vi "Panel.vi"(11 "StringPanel in":refnum<class "StringPanel.lvclass">) -> ()   [LabVIEW 2020, in "Conditum-Tools.lvlib" / "StringPanel.lvclass"]
uses:
  StringPanel.lvclass
  C:/dev/lv20CE/lv-conditum-tools/Conditum-Tools/ColumnPanel/ColumnPanel.lvclass
  C:/Program Files (x86)/National Instruments/LabVIEW 2020/vi.lib/IlluminatedG/IG OOPanel/OOPanel/Panel/Panel.lvclass
  ColumnPanel/Common Items.ctl
  <vilib>/IlluminatedG/IG OOPanel/OOPanel/Panel/Basic UI State.ctl
  StringPanel.lvclass/StringPanel.ctl
  Conditum-Clone/Columns/Type/Type.lvclass/Type.ctl
  Conditum-Clone/Columns/String/String Definition.ctl
  Conditum-Clone/Columns/Type/Definition.ctl
  Conditum-Clone/Attributes.ctl
  Conditum-Clone/Columns/String/Definition.ctl
  18b06730-9059-4579-972d-706e62b01def.vi
  Conditum-Clone/Columns/String/String.lvclass
  C:/dev/lv20CE/lv-conditum-tools/Conditum-Clone/Columns/Type/Type.lvclass
  Conditum-Clone/Columns/Type/Type.lvclass
  <vilib>/IlluminatedG/IG OOPanel/OOPanel/Panel/Panel.lvclass
  ColumnPanel/ColumnPanel.lvclass
  Conditum-Clone/Conditu2.lvlib
  <vilib>/IlluminatedG/IG OOPanel/OOPanel/OOPanel.lvlib
  C:/Program Files (x86)/National Instruments/LabVIEW 2020/vi.lib/IlluminatedG/IG OOPanel/OOPanel/ArrayPanel/ArrayPanel.lvclass
  C:/dev/lv20CE/lv-conditum-tools/Conditum-Tools/StringPanel/StringPanel.lvclass
panel:
  in  "Max Length":i32=255
  in  "Default Value":string
  in  "Common Items":T1
  # "String"
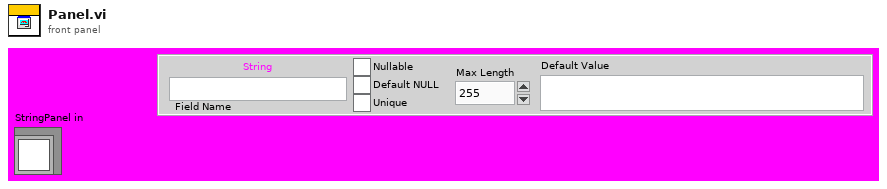
[diagram p1: front panel]
types:
  T1 = typedef "Conditum-Tools.lvlib/ColumnPanel.lvclass/Common Items.ctl" = cluster{"Name":string, "Nullable":bool, "Default NULL":bool, "Unique":bool}
  T2 = typedef "OOPanel.lvlib/Panel.lvclass/Basic UI State.ctl" = enum16{"Init", "Run", "Close"}
  T3 = typedef "Conditu2.lvlib/Columns.lvlib/String.lvclass/String Definition.ctl" = cluster{"Type":T4, "Attributes":T5, "String":T6}
  T4 = typedef "Conditu2.lvlib/Columns.lvlib/Type.lvclass/Definition.ctl" = cluster{"Name":string, "Nullable":bool, "Default NULL":bool}
  T5 = typedef "Conditu2.lvlib/Attributes.ctl" = cluster{"Primary Key":bool, "Unique":bool, "Foreign Key":bool, "Auto Increment":bool}
  T6 = typedef "Conditu2.lvlib/Columns.lvlib/String.lvclass/Definition.ctl" = cluster{"Default":string, "Length":i32}
  T7 = typedef "OOPanel.lvlib/Panel.lvclass/Panel Events.ctl" = cluster{"Visbility":refnum<user-event>, "Close":refnum<user-event>}
  T8 = typedef "Conditum-Tools.lvlib/ColumnPanel.lvclass/Events.ctl" = cluster{"Update":refnum<user-event>, "Value":refnum<user-event>, "Valid":refnum<user-event>, "Highlight":refnum<user-event>}
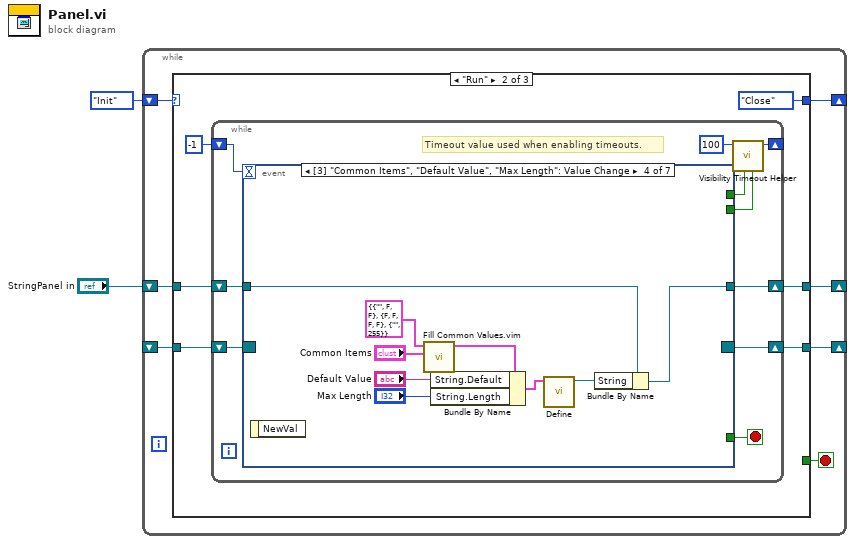
[diagram p0: block diagram]
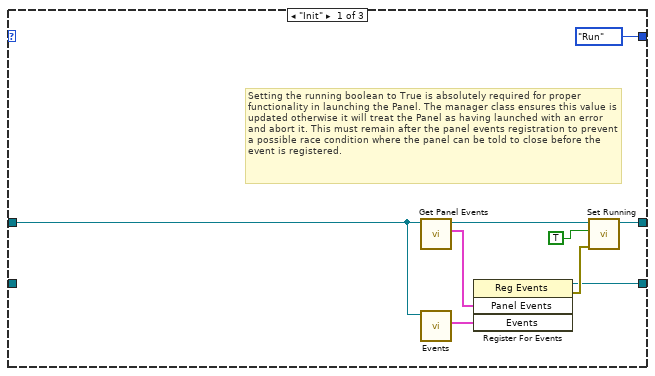
[diagram p2: hidden frame]
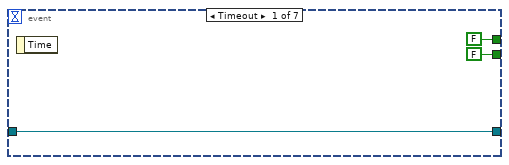
[diagram p3: hidden frame]
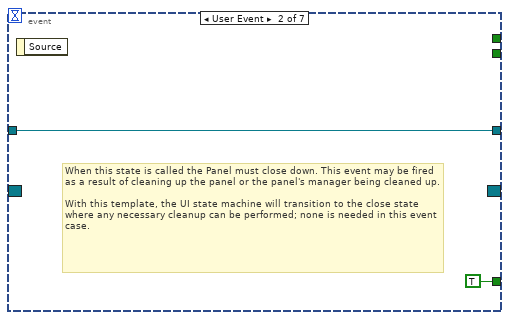
[diagram p4: hidden frame]
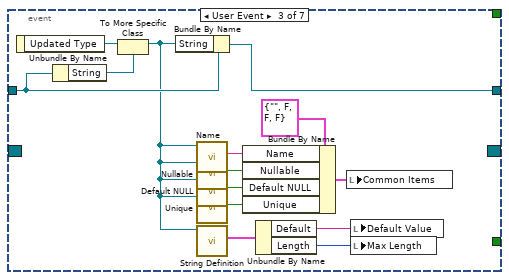
[diagram p5: hidden frame]
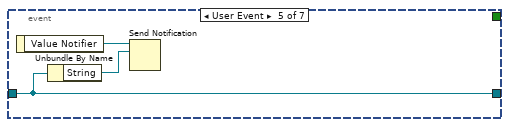
[diagram p6: hidden frame]
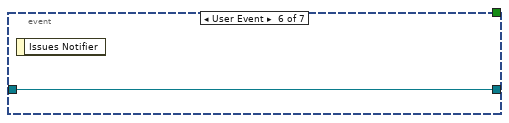
[diagram p7: hidden frame]
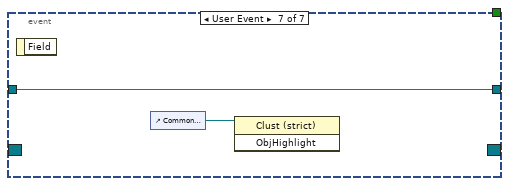
[diagram p8: hidden frame]
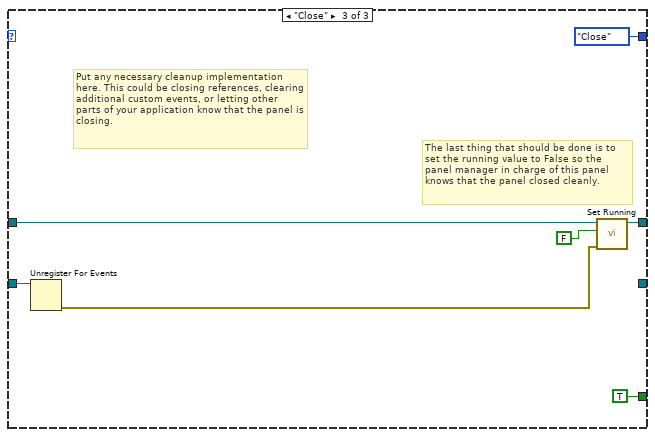
[diagram p9: hidden frame]
diagram:
  n1 = while {
    shift-right: [w8] -> _
    shift-left: _ -> [w9]
    shift-right: [w6] -> _
    shift-left: Basic_UI_State."Init" ("Basic UI State") -> [w7]
    shift-right: [w4] -> _
    shift-left: "StringPanel in" -> [w3]
    stop <- w5 stop-if-true
    n2 = case shown="\"Run\"" w7 {
      tunnel: w9 -> [_ w24 w71]
      tunnel: [w15 w22 _] -> w8
      tunnel: [Basic_UI_State."Run" ("Basic UI State") Basic_UI_State."Close" ("Basic UI State") Basic_UI_State."Close" ("Basic UI State")] -> w6
      tunnel: [_ _ TRUE] -> w5
      tunnel: [w14 w19 w69] -> w4
      tunnel: w3 -> [w10 w20 w70]
      frame "Init" {
        # "Setting the running boolean to True is absolutely required for proper functionality in launching the Panel. The manager class ensures this value is updated otherwise it will treat the Panel as having launched with an error and abort it. This must remain after the panel events registration to prevent a possible race condition where the panel can be told to close before the event is registered."
        n3 = call <vilib>:"Get Panel Events.vi"("Panel in"=w10) -> ("Panel Events"=w12:T7, "Panel out"=w13:refnum<class "StringPanel.lvclass">)  [unwired: 8 in, 1 out]
        n4 = call "Events.vi"("ColumnPanel in"=w10) -> ("Events"=w11:T8)  [unwired: 10 in]
        n5 = register-events(w12, w11) -> (reference out=w15:refnum<event-registration>, error out=w17:errorcluster)  [unwired: 2 in]
        n6 = call <vilib>:"Set Running.vi"("error in (no error)"=w17, "Running"=TRUE, "Panel in"=w13) -> ("Panel out"=w14:refnum<class "StringPanel.lvclass">)  [unwired: 7 in, 1 out]
      }
      frame "Run" {
        n7 = while {
          shift-right: [w30] -> w22
          shift-left: w24 -> [w31]
          shift-right: [w33] -> _
          shift-left: -1 ("Timeout") -> [w32]
          shift-right: [w25] -> w19
          shift-left: w20 -> [w26]
          stop <- w27 stop-if-true
          # "Timeout value used when enabling timeouts."
          n8 = event shown="[3] \"Common Items\", \"Default Value\", \"Max Length\": Value Change" {
            selector: w31 -> [_ _ _ _ _ _ _]
            dyn-events: [_ _ _ _ _ _ _] -> w30
            timeout: w32 -> [_ _ _ _ _ _ _]
            tunnel: [FALSE _ _ _ _ _ _] -> w29
            tunnel: [FALSE _ _ _ _ _ _] -> w28
            tunnel: [_ TRUE _ _ _ _ _] -> w27
            tunnel: w26 -> [w35 w38 w51 w57 w65 w66 w68]
            tunnel: [w35 w38 w52 w58 w65 w66 w68] -> w25
            event Timeout {
              n9 = event-data() -> ()  [unwired: 1 in, 1 out]
            }
            event User Event {
              # "When this state is called the Panel must close down. This event may be fired as a result of cleaning up the panel or the panel's manager being cleaned up.\n\nWith this template, the UI state machine will transition to the close state where any necessary cleanup can be performed; none is needed in this event case."
              n10 = event-data() -> ()  [unwired: 1 in, 1 out]
            }
            event User Event {
              n11 = event-data() -> ("Updated Type"=w53:refnum<class "Type.lvclass">)  [unwired: 1 in]
              n12 = Unbundle By Name(w51) -> ("String"=w50:refnum<class "String.lvclass">)
              n13 = To More Specific Class(target class=w50, reference=w53) -> (specific class reference=w43:refnum<class "String.lvclass">)  [unwired: 1 in, 1 out]
              n14 = Bundle By Name(cluster=w51, "String"=w43) -> (w52:refnum<class "StringPanel.lvclass">)
              n15 = call "Name.vi"("Type in"=w43) -> ("Table Name"=w47:string)  [unwired: 10 in]
              n16 = call "Nullable.vi"("Type in"=w43) -> ("Nullable"=w46:bool)  [unwired: 10 in]
              n17 = call "Default NULL.vi"("Type in"=w43) -> ("Default NULL"=w45:bool)  [unwired: 10 in]
              n18 = call "Unique.vi"("Type in"=w43) -> ("Unique"=w44:bool)  [unwired: 10 in]
              n19 = call "String Definition.vi"("String in"=w43) -> ("Definition"=w42:T6)  [unwired: 10 in]
              n20 = Bundle By Name(cluster=T1 {"Name"="", "Nullable"=FALSE, "Default NULL"=FALSE, "Unique"=FALSE} ("Common Items"), "Name"=w47, "Nullable"=w46, "Default NULL"=w45, "Unique"=w44) -> (w48:T1)
              n21 = Unbundle By Name(w42) -> ("Default"=w40:string, "Length"=w41:i32)
              n22 = local write "Common Items"(w48) -> ()
              n23 = local write "Default Value"(w40) -> ()
              n24 = local write "Max Length"(w41) -> ()
            }
            event "Default Value", "Max Length": Value Change {
              n25 = event-data() -> ()  [unwired: 1 in, 1 out]
              n26 = call "Fill Common Values.vim"("Common Items"="Common Items", "Init Data Type"=T3 {"Type"={"Name"="", "Nullable"=FALSE, "Default NULL"=FALSE}, "Attributes"={"Primary Key"=FALSE, "Unique"=FALSE, "Foreign Key"=FALSE, "Auto Increment"=FALSE}, "String"={"Default"="", "Length"=255}} ("Init Data")) -> ("Init Data"=w55:T3)  [unwired: 9 in]
              n27 = Bundle By Name(cluster=w55, "String.Default"="Default Value", "String.Length"="Max Length") -> (w61:T3)
              n28 = call "Define.vi"("Definition"=w61) -> ("String out"=w59:refnum<class "String.lvclass">)  [unwired: 10 in]
              n29 = Bundle By Name(cluster=w57, "String"=w59) -> (w58:refnum<class "StringPanel.lvclass">)
            }
            event User Event {
              n30 = event-data() -> ("Value Notifier"=w64:refnum<notifier>)  [unwired: 1 in]
              n31 = Unbundle By Name(w65) -> ("String"=w63:refnum<class "String.lvclass">)
              n32 = Send Notification(notification=w63, notifier=w64) -> ()  [unwired: 1 in, 2 out]
            }
            event User Event {
              n33 = event-data() -> ()  [unwired: 1 in, 1 out]
            }
            event User Event {
              n34 = event-data() -> ()  [unwired: 1 in, 1 out]
              n35 = control-ref of="Common Items"() -> (w67:refnum<vi>)
              n36 = invoke class="Clust (strict)" method="ObjHighlight"(reference=w67) -> ()  [unwired: 2 in, 3 out]
            }
          }
          n37 = call <vilib>:"Visibility Timeout Helper.vi"("Update?"=w28, "Use Timeout?"=w29, "Visible Timeout mS"=100) -> ("Timeout"=w33:i32)  [unwired: 8 in]
        }
      }
      frame "Close" {
        # "Put any necessary cleanup implementation here. This could be closing references, clearing additional custom events, or letting other parts of your application know that the panel is closing."
        # "The last thing that should be done is to set the running value to False so the panel manager in charge of this panel knows that the panel closed cleanly."
        n38 = Unregister For Events(event registration refnum=w71) -> (error out=w73:errorcluster)  [unwired: 1 in]
        n39 = call <vilib>:"Set Running.vi"("error in (no error)"=w73, "Running"=FALSE, "Panel in"=w70) -> ("Panel out"=w69:refnum<class "StringPanel.lvclass">)  [unwired: 7 in, 1 out]
      }
    }
  }
